vi "Localize VIs.vi"(6 "Additional Languages [English]":string[](array[string])=["English"], 8 "error in (no error)":errorcluster, 9 "Current VI Language (English)":string="English", 10 "Dictionary Path":path, 11 "VIs in":refnum<vi>[](array[refnum])) -> (0 "error out":errorcluster)   [LabVIEW 2019]
doc: "Writes VI text to a new JSON dictionary file. The file will need to be updated to include the additional languages."
panel:
  out "Text Written (for debug)":string
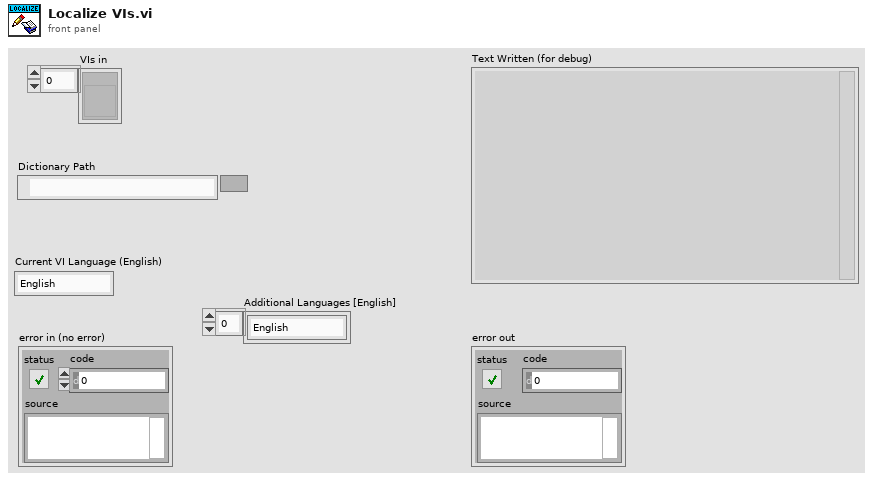
[diagram p1: front panel]
types:
  T1 = typedef "Dictionary--Cluster.ctl" = cluster{"Format Version":string, "Languages":T2[], "Phrase Dictionary":T3[]}
  T2 = typedef "Font -- Cluster.ctl" = cluster{"Language":string, "Font":string, "Color":string}
  T3 = typedef "Phrase Dictionary Entry -- Cluster.ctl" = cluster{"Key":string, "Phrases":string[]}
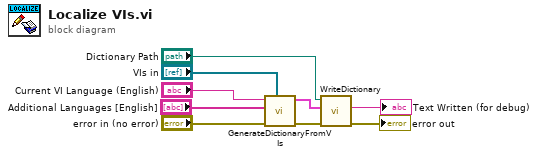
[diagram p0: block diagram]
diagram:
  n1 = call "GenerateDictionaryFromVIs.vi"("VIs in"="VIs in", "error in (no error)"="error in (no error)", "Additional Languages [English]"="Additional Languages [English]", "Current VI Language (English)"="Current VI Language (English)") -> ("error out"=w4:errorcluster, "Localization"=w3:T1)  [unwired: 6 in]
  n2 = call "WriteDictionary.vi"("error in (no error)"=w4, "Localization"=w3, "Dictionary Path"="Dictionary Path") -> ("error out"=→"error out":errorcluster, "CSV String"=→"Text Written (for debug)":string)  [unwired: 6 in, 1 out]
